vi "Lightning Begin.vi"() -> (0 "error out":errorcluster)   [LabVIEW 2014]
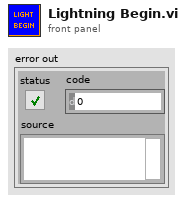
[diagram p1: front panel]
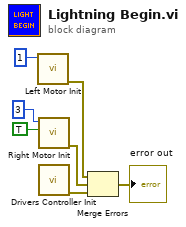
[diagram p0: block diagram]
diagram:
  n1 = call "Left Motor Init.vi"("CAN Id"=u8 1) -> ("error out"=w3:errorcluster)  [unwired: 10 in]
  n2 = call "Right Motor Init.vi"("Invert (default false)"=TRUE, "CAN Id"=u8 3) -> ("error out"=w4:errorcluster)  [unwired: 9 in]
  n3 = call "Drivers Controller Init.vi"() -> ("error out"=w1:errorcluster)  [unwired: 11 in]
  n4 = Merge Errors(w3, w4, w1) -> (→"error out":errorcluster)
